vi "MJG_StageHoming_v1.vi"(8 "error in":errorcluster, 11 "FPGA VI Reference In":refnum<k20>) -> (0 "error out":errorcluster, 2 "XYZ Offsets [enc cnts]":i32[](array[numeric]), 3 "FPGA VI Reference Out":refnum<k20>)   [LabVIEW 2016]
uses:
  IRISSoft LV2016/Subsystems/Global Variables.vi
  <vilib>/Utility/error.llb/Error Cluster From Error Code.vi
  <vilib>/rvi/errors/niLvFpgaAdjustHostInterfaceError.vi
  <vilib>/rvi/interface/nirviReadWriteControl/nirviReadWriteControl.xnode
  IRISSoft LV2016/FPGA Bitfiles/PhantomControlPI_FPGATarget_QuadCtr2_E2412E44.lvbitx
  IRISSoft LV2016/IRISS_FPGA_IO.vi
  NiFpgaLv.dll
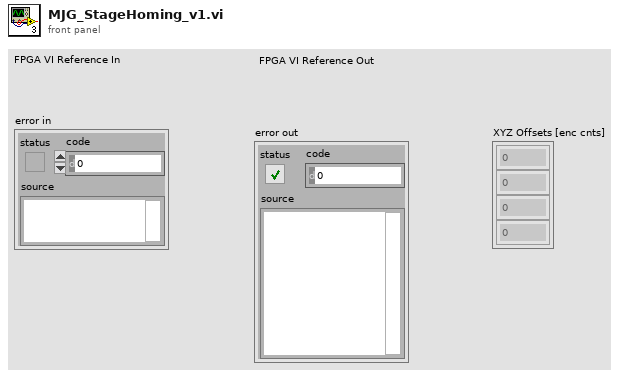
[diagram p1: front panel]
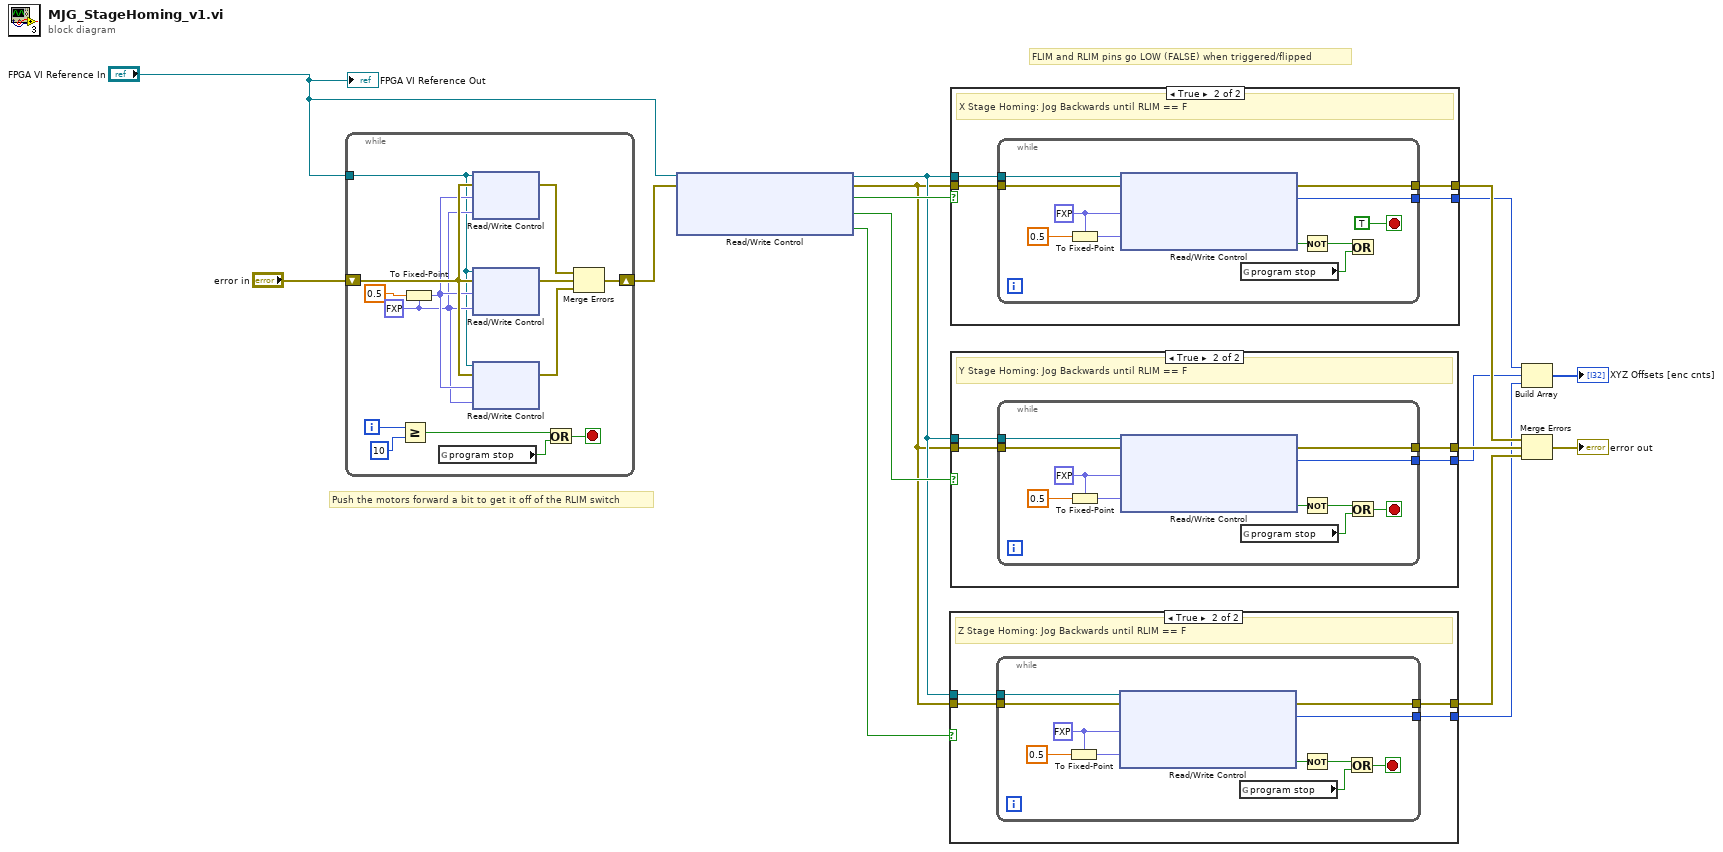
[diagram p0: block diagram]
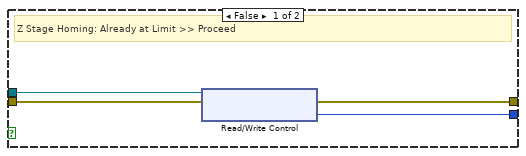
[diagram p2: hidden frame]
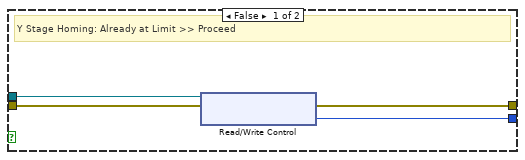
[diagram p3: hidden frame]
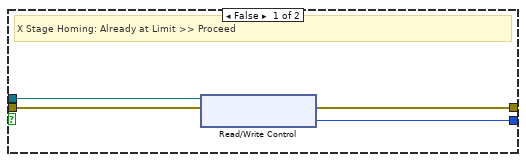
[diagram p4: hidden frame]
diagram:
  # "Push the motors forward a bit to get it off of the RLIM switch"
  # "FLIM and RLIM pins go LOW (FALSE) when triggered/flipped"
  n1 = while {
    shift-right: [w25] -> w2
    shift-left: "error in" -> [w26]
    tunnel: "FPGA VI Reference In" -> [w17]
    i -> [w24]
    stop <- w20 stop-if-true
    w18 = fxp<+,32,0> 0.0 ("X PWM 2")
    n2 = Greater Or Equal?(x=w24, y=10) -> (x >= y?=w22:bool)
    n3 = To Fixed-Point(fixed-point type=w18, number=0.5 ("y")) -> (fixed-point=w19:fxp<+,32,0>)
    n4 = global read "Global Variables.vi" "program stop"() -> (w21:bool)
    n5 = xnode "Read/Write Control"("FPGA VI Reference In"=w17, "error in"=w26, "X PWM 1"=w19, "X PWM 2"=w18) -> ("error out"=w29:errorcluster)  [unwired: 1 out]
    n6 = xnode "Read/Write Control"("FPGA VI Reference In"=w17, "error in"=w26, "Y PWM 1"=w19, "Y PWM 2"=w18) -> ("error out"=w28:errorcluster)  [unwired: 1 out]
    n7 = xnode "Read/Write Control"("FPGA VI Reference In"=w17, "error in"=w26, "Z PWM 1"=w19, "Z PWM 2"=w18) -> ("error out"=w27:errorcluster)  [unwired: 1 out]
    n8 = Or(x=w22, y=w21) -> (x .or. y?=w20:bool)
    n9 = Merge Errors(w29, w28, w27) -> (w25:errorcluster)
  }
  n10 = xnode "Read/Write Control"("FPGA VI Reference In"="FPGA VI Reference In", "error in"=w2) -> ("FPGA VI Reference Out"=w13:refnum<k20>, "error out"=w12:errorcluster, "X Stage RLIM (CONN2/DIO32)"=w16:bool, "Y Stage RLIM (CONN2/DIO35)"=w15:bool, "Z Stage RLIM (CONN2/DIO38)"=w14:bool)
  n11 = case shown="True" w14 {
    tunnel: w13 -> [w33 w38]
    tunnel: w12 -> [w34 w37]
    tunnel: [w32 w36] -> w8
    tunnel: [w31 w35] -> w5
    frame False {
      # "Z Stage Homing: Already at Limit >> Proceed"
      n12 = xnode "Read/Write Control"("FPGA VI Reference In"=w33, "error in"=w34) -> ("error out"=w32:errorcluster, "Z Stage Enc Count"=w31:i32)  [unwired: 1 out]
    }
    frame True {
      # "Z Stage Homing: Jog Backwards until RLIM == F"
      n13 = while {
        tunnel: w38 -> [w44]
        tunnel: w37 -> [w43]
        tunnel: [w42] -> w36
        tunnel: [w39] -> w35
        stop <- w48 stop-if-true
        w46 = fxp<+,32,0> 0.0 ("X PWM 2")
        n14 = To Fixed-Point(fixed-point type=w46, number=0.5 ("y")) -> (fixed-point=w45:fxp<+,32,0>)
        n15 = xnode "Read/Write Control"("FPGA VI Reference In"=w44, "error in"=w43, "Z PWM 1"=w46, "Z PWM 2"=w45) -> ("error out"=w42:errorcluster, "Z Stage Enc Count"=w39:i32, "Z Stage RLIM (CONN2/DIO38)"=w41:bool)  [unwired: 1 out]
        n16 = global read "Global Variables.vi" "program stop"() -> (w47:bool)
        n17 = Not(x=w41) -> (.not. x?=w40:bool)
        n18 = Or(x=w40, y=w47) -> (x .or. y?=w48:bool)
      }
    }
  }
  n19 = case shown="True" w16 {
    tunnel: w13 -> [w52 w57]
    tunnel: w12 -> [w53 w56]
    tunnel: [w51 w55] -> w10
    tunnel: [w50 w54] -> w7
    frame False {
      # "X Stage Homing: Already at Limit >> Proceed"
      n20 = xnode "Read/Write Control"("FPGA VI Reference In"=w52, "error in"=w53) -> ("error out"=w51:errorcluster, "X Stage Enc Count"=w50:i32)  [unwired: 1 out]
    }
    frame True {
      # "X Stage Homing: Jog Backwards until RLIM == F"
      n21 = while {
        tunnel: w57 -> [w64]
        tunnel: w56 -> [w63]
        tunnel: [w62] -> w55
        tunnel: [w59] -> w54
        stop <- TRUE stop-if-true
        w66 = fxp<+,32,0> 0.0 ("X PWM 2")
        n22 = To Fixed-Point(fixed-point type=w66, number=0.5 ("y")) -> (fixed-point=w65:fxp<+,32,0>)
        n23 = xnode "Read/Write Control"("FPGA VI Reference In"=w64, "error in"=w63, "X PWM 1"=w66, "X PWM 2"=w65) -> ("error out"=w62:errorcluster, "X Stage Enc Count"=w59:i32, "X Stage RLIM (CONN2/DIO32)"=w61:bool)  [unwired: 1 out]
        n24 = global read "Global Variables.vi" "program stop"() -> (w67:bool)
        n25 = Not(x=w61) -> (.not. x?=w60:bool)
        n26 = Or(x=w60, y=w67) -> ()  [unwired: 1 out]
      }
    }
  }
  n27 = case shown="True" w15 {
    tunnel: w13 -> [w71 w76]
    tunnel: w12 -> [w72 w75]
    tunnel: [w70 w74] -> w9
    tunnel: [w69 w73] -> w6
    frame False {
      # "Y Stage Homing: Already at Limit >> Proceed"
      n28 = xnode "Read/Write Control"("FPGA VI Reference In"=w71, "error in"=w72) -> ("error out"=w70:errorcluster, "Y Stage Enc Count"=w69:i32)  [unwired: 1 out]
    }
    frame True {
      # "Y Stage Homing: Jog Backwards until RLIM == F"
      n29 = while {
        tunnel: w76 -> [w82]
        tunnel: w75 -> [w81]
        tunnel: [w80] -> w74
        tunnel: [w77] -> w73
        stop <- w86 stop-if-true
        w84 = fxp<+,32,0> 0.0 ("X PWM 2")
        n30 = To Fixed-Point(fixed-point type=w84, number=0.5 ("y")) -> (fixed-point=w83:fxp<+,32,0>)
        n31 = xnode "Read/Write Control"("FPGA VI Reference In"=w82, "error in"=w81, "Y PWM 1"=w84, "Y PWM 2"=w83) -> ("error out"=w80:errorcluster, "Y Stage Enc Count"=w77:i32, "Y Stage RLIM (CONN2/DIO35)"=w79:bool)  [unwired: 1 out]
        n32 = global read "Global Variables.vi" "program stop"() -> (w85:bool)
        n33 = Not(x=w79) -> (.not. x?=w78:bool)
        n34 = Or(x=w78, y=w85) -> (x .or. y?=w86:bool)
      }
    }
  }
  n35 = Build Array(w7, w6, w5) -> (→"XYZ Offsets [enc cnts]":i32[])
  n36 = Merge Errors(w10, w9, w8) -> (→"error out":errorcluster)
  "FPGA VI Reference Out" <- "FPGA VI Reference In"
